vi "DAQ_BlueSteel.vi"() -> ()   [LabVIEW 2016]
uses:
  Control 1.ctl
  <vilib>/DAQmx/write.llb/DAQmx Write (Digital 1D Bool 1Chan 1Samp).vi
  <vilib>/DAQmx/create/channels.llb/DAQmx Create Channel (DO-Digital Output).vi
  <vilib>/DAQmx/miscellaneous.llb/DAQmx Fill In Error Info.vi
  <vilib>/DAQmx/create/channels.llb/DAQmx Create Channel (CO-Pulse Generation-Frequency).vi
  <vilib>/DAQmx/configure/timing.llb/DAQmx Timing (Implicit).vi
  <resource>/objmgr/daqmx.rc
panel:
  out "Ignition":bool
  out "Pump":bool
  out "Record Status":string
  out "TCp-3P Status":bool
  out "TCp-3P":dbl
  out "FM-F Status":bool
  out "FM-F":dbl
  in  "Record":bool
  out "Recording":bool
  out "Solenoid\nStatus":bool[](array[boolean])
  in  "Tab Control":enum32{"Operations", "Testing", "Parameters"}(tab)
  in  "Firing Mode":bool
  in  "Enable Fire Button":bool
  in  "Fuel Arm":bool
  in  "ARM":bool
  in  "ABORT":bool
  out "Arm Indicator":bool
  out "Fuel Arm Indicator 10":bool
  in  "Pressurize":bool
  out "Engine State":string
  out "SAFE":bool
  in  "FIRE":bool
  in  "F Purge":bool
  in  "O Purge":bool
  out "Ox Purged":bool
  out "Fuel Purged":bool
  in  "Depressurize":bool
  out "Fill Volume Bar":dbl(slide) max=258.9 scale=0.0..258.9
  out "Fill Volume (in^3)":dbl
  in  "Manual Fill Reset":bool
  in  "Fuel Prime":bool
  in  "Igniter Prime":bool
  in  "Finish Filling":bool
  in  "Enable Fill Reset":bool
  out "Filled":bool
  in  "Fuel Purge":bool
  in  "Oxygen Purge":bool
  in  "Warning Override":bool
  in  "Spark Safety":bool
  in  "Safety Override":bool[](array[boolean])
  in  "Pump Test":bool
  in  "Spark Test":bool
  in  "NC-P":bool
  in  "NO-P":bool
  in  "NC-F":bool
  in  "NC-O":bool
  in  "NC-IF":bool
  in  "NC-IO":T1
  in  "Parameters":dbl[](array[numeric])
  in  "Max Volume (in^3)":dbl
  in  "Fill Rate (in^3/s)":dbl
  out "PT-TI Status":bool
  out "PT-TI":dbl
  out "PT-IO Status":bool
  out "PT-IO":dbl
  out "FM-O Status":bool
  out "FM-O":dbl
  out "PT-3P Status":bool
  out "PT-3P":dbl
  out "PT-2E Status":bool
  out "PT-2E":dbl
  out "PT-1E Status":bool
  out "PT-1E":dbl
  out "PT-2P Status":bool
  out "PT-2P":dbl
  out "PT-1P Status":bool
  out "PT-1P":dbl
  out "PT-3O Status":bool
  out "PT-3O":dbl
  out "PT-2O Status":bool
  out "PT-2O":dbl
  out "PT-1O Status":bool
  out "PT-1O":dbl
  out "PT-IF Status":bool
  out "PT-IF":dbl
  out "PT-3F Status":bool
  out "PT-3F":dbl
  out "PT-2F Status":bool
  out "PT-2F":dbl
  out "PT-1F Status":bool
  out "PT-1F":dbl
  out "PT-L Status":bool
  out "PT-L":dbl
  out "LC-1E Status":bool
  out "LC-1E":dbl
  out "TCp-2P Status":bool
  out "TCp-2P":dbl
  out "TCp-1P Status":bool
  out "TCp-1P":dbl
  out "TCp-TI Status":bool
  out "TCp-TI":dbl
  out "TCp-2F Status":bool
  out "TCp-2F":dbl
  out "TCp-1F Status":bool
  out "TCp-1F":dbl
  out "TCw-4E Status":bool
  out "TCw-4E":dbl
  out "TCw-3E Status":bool
  out "TCw-3E":dbl
  out "TCw-2E Status":bool
  out "TCw-2E":dbl
  out "TCw-1E Status":bool
  out "TCw-1E":dbl
  out "TCp-3O Status":bool
  out "TCp-3O":dbl
  out "TCp-2O Status":bool
  out "TCp-2O":dbl
  out "TCp-1O Status":bool
  out "TCp-1O":dbl
  # "Red warnings are based on the sensor warning chart in the DAQ project folder on The LPL Drive. A warning will cause an\nautomatic abort on the Operations pane.\n\nThese warnings do not prevent the operation of switches in the Testing pane."
  # "Thermocouples  (F)"
  # "Load Cells (lbf)"
  # "Flow Meters (kg/s)"
  # "Pressure Transducers (psi)"
  # "NC-P"
  # "NO-P"
  # "NC-F"
  # "NC-O"
  # "NC-IF"
  # "NC-IO"
  # "Hot\nFire"
  # "Igniter\nTest"
  # "WARNING: Follow fill procedures to ensure proper\npriming and to avoid fuel waste."
  # "Warning override prevents automatic aborts when\nred flags are active on any sensor readouts."
  # "Safety override is required when PTs on either side of the valve \nread > 100 psid."
  # "Fill Parameters"
  # "Pressurisation P tolerance lower limit (psi)"
  # "Pressurisation P tolerance upper limit (psi)"
  # "Fuel delay (secs)"
  # "Ox delay (secs)"
  # "Spark delay (secs)"
  # "Ignitor pressure threshold (psi)"
  # "Combustion pressure threshold (psi)"
  # "Ignitor run time (secs)"
  # "Engine run time (secs)"
  # "Fuel line pressure threshold (psi)"
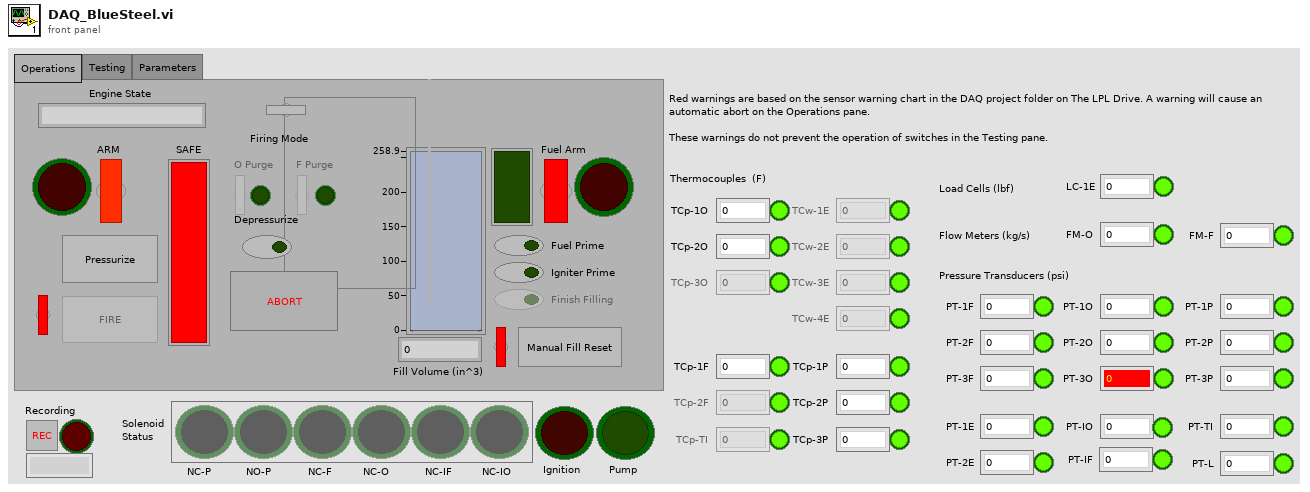
[diagram p1: front panel]
types:
  T1 = typedef "Control 1.ctl" = bool
  T2 = enum8{"Enabled", "Disabled", "Disabled and Grayed Out"}
  T3 = cluster{"[0]":dbl, "[1]":dbl, "[2]":dbl, "[3]":dbl, "[4]":dbl, "[5]":dbl, "[6]":dbl, "[7]":dbl, "[8]":dbl}
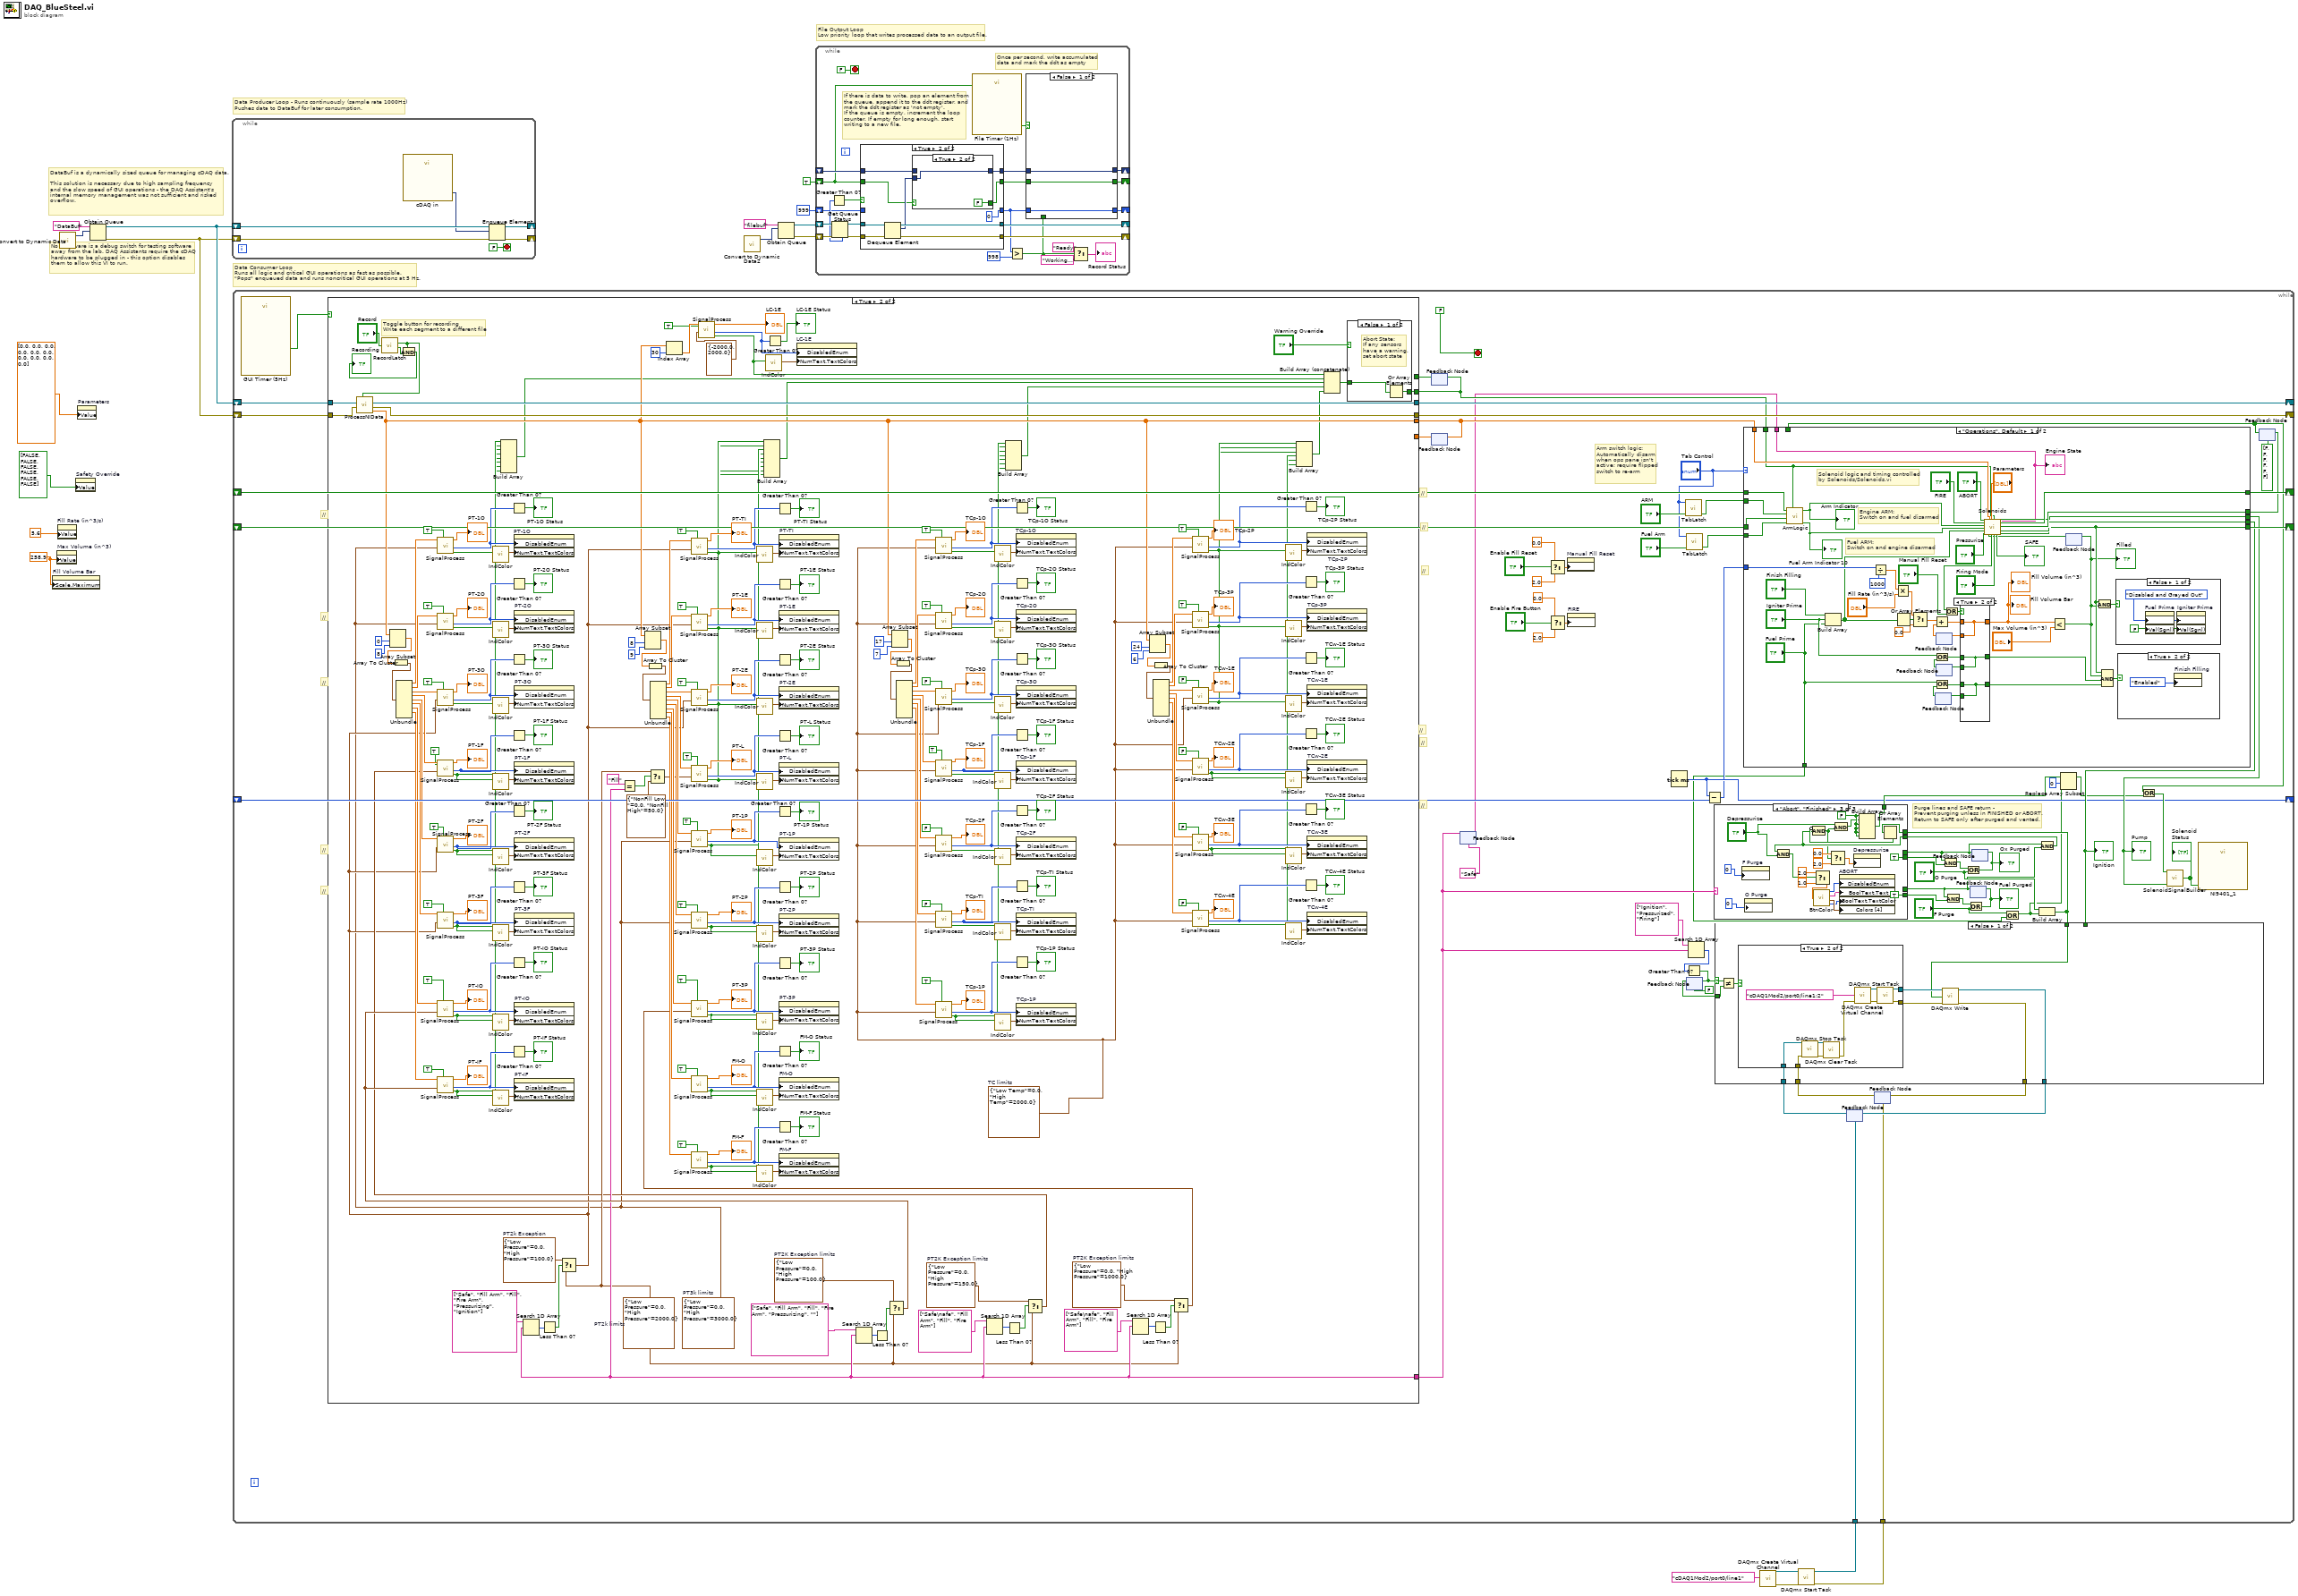
[diagram p0: block diagram]
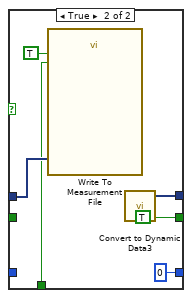
[diagram p2: hidden frame]
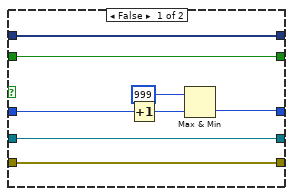
[diagram p3: hidden frame]
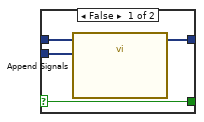
[diagram p4: hidden frame]
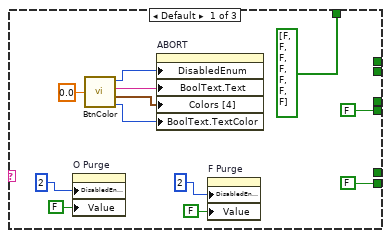
[diagram p5: hidden frame]
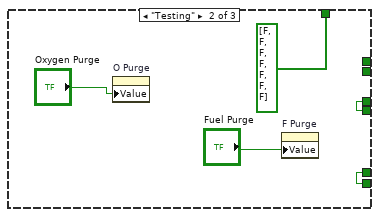
[diagram p6: hidden frame]
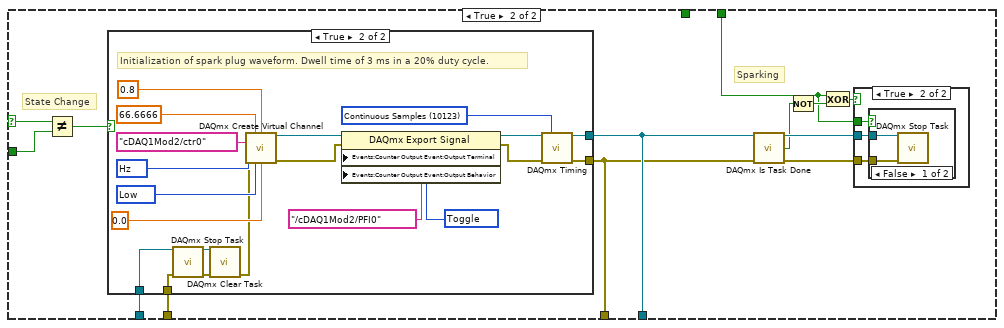
[diagram p8: hidden frame]
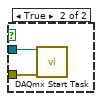
[diagram p10: hidden frame]
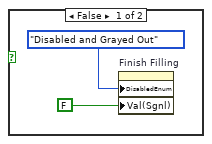
[diagram p12: hidden frame]
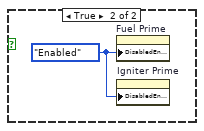
[diagram p13: hidden frame]
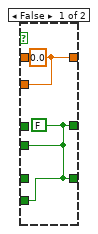
[diagram p14: hidden frame]
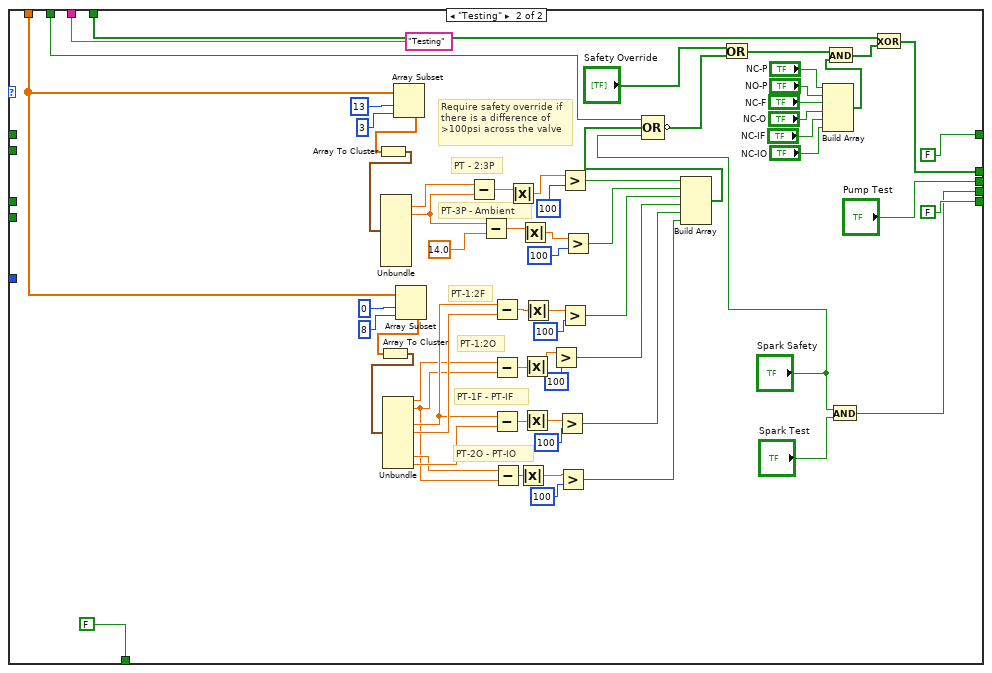
[diagram p15: hidden frame]
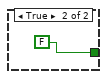
[diagram p17: hidden frame]
diagram:
  w1 = 258.9
  # "File Output Loop\nLow priority loop that writes processed data to an output file."
  # "Data Consumer Loop\nRuns all logic and critical GUI operations as fast as possible.\n\"Pops\" enqueued data and runs noncritical GUI operations at 5 Hz."
  # "No Hardware is a debug switch for testing software\naway from the lab. DAQ Assistants require the cDAQ\nhardware to be plugged in - this option disables \nthem to allow this VI to run."
  # "Data Producer Loop - Runs continuously (sample rate 1000Hz)\nPushes data to DataBuf for later consumption."
  # "DataBuf is a dynamically sized queue for managing cDAQ data.\n\nThis solution is necessary due to high sampling frequency \nand the slow speed of GUI operations - the DAQ Assistant's\ninternal memory management was not sufficient and risked\noverflow."
  n1 = property on="Fill Volume Bar" class="Slide (strict)"("Scale.Maximum"=w1) -> ()  [unwired: 2 in, 2 out]
  n2 = property on="Max Volume (in^3)" class="DigNum (strict)"("Value"=w1) -> ()  [unwired: 2 in, 2 out]
  n3 = property on="Fill Rate (in^3/s)" class="DigNum (strict)"("Value"=5.6) -> ()  [unwired: 2 in, 2 out]
  n4 = call "Convert to Dynamic Data"() -> ("Dynamic Data Type"=w18:dynamicdata)  [unwired: 4 in]
  n5 = property on="Safety Override" class="Arr (strict)"("Value"=bool[] [FALSE, FALSE, FALSE, FALSE, FALSE, FALSE]) -> ()  [unwired: 2 in, 2 out]
  n6 = property on="Parameters" class="Arr (strict)"("Value"=dbl[] [0.0, 0.0, 0.0, 0.0, 0.0, 0.0, 0.0, 0.0, 0.0, 0.0]) -> ()  [unwired: 2 in, 2 out]
  n7 = Obtain Queue(name (unnamed)="DataBuf", element data type=w18) -> (queue out=w17:refnum<queue>, error out=w16:errorcluster)  [unwired: 3 in, 1 out]
  n8 = while {
    shift-right: [w22] -> _
    shift-left: w16 -> [w23]
    shift-right: [w24] -> _
    shift-left: w17 -> [w25]
    stop <- FALSE stop-if-true
    n9 = call "cDAQ in"() -> ("data"=w20:dynamicdata)  [unwired: 16 in, 3 out]
    n10 = Enqueue Element(queue=w25, element=w20, error in (no error)=w23) -> (queue out=w24:refnum<queue>, error out=w22:errorcluster)  [unwired: 1 in, 1 out]
  }
  n11 = call "Convert to Dynamic Data2"() -> ("Dynamic Data Type"=w14:dynamicdata)  [unwired: 4 in]
  n12 = Obtain Queue(name (unnamed)="filebuf", element data type=w14) -> (queue out=w13:refnum<queue>, error out=w12:errorcluster)  [unwired: 3 in, 1 out]
  n13 = while {
    shift-right: [w48] -> _
    shift-left: w12 -> [w40]
    shift-right: [w49] -> _
    shift-left: w13 -> [w41]
    shift-right: [w46] -> _
    shift-left: _ -> [w47]
    shift-right: [w45] -> _
    shift-left: TRUE -> [w34]
    shift-right: [w32] -> _
    shift-left: 999 -> [w33]
    stop <- FALSE stop-if-true
    # "If there is data to write, pop an element from\nthe queue, append it to the ddt register, and\nmark the ddt register as 'not empty'.\nIf the queue is empty, increment the loop\ncounter. If empty for long enough, start\nwriting to a new file."
    # "Once per second, write accumulated\ndata and mark the ddt as empty"
    n14 = Get Queue Status(queue=w41, error in (no error)=w40) -> (queue out=w43:refnum<queue>, error out=w42:errorcluster, # elements in queue=w38:i32)  [unwired: 1 in, 5 out]
    n15 = Greater Than 0?(x=w38) -> (x > 0?=w39:bool)
    n16 = case shown="True" w39 {
      tunnel: w43 -> [w65 w76]
      tunnel: w42 -> [w64 w75]
      tunnel: [w65 w74] -> w49
      tunnel: [w64 w73] -> w48
      tunnel: [w66 w72] -> w37
      tunnel: w47 -> [w66 w70]
      tunnel: w34 -> [w63 w69]
      tunnel: [w63 w68] -> w36
      tunnel: w33 -> [w62 _]
      tunnel: [w59 0] -> w28
      frame False {
        n17 = Increment(x=w62) -> (x+1=w61:i32)
        n18 = Max & Min(x=999, y=w61) -> (min(x,y)=w59:i32)  [unwired: 1 out]
      }
      frame True {
        n19 = Dequeue Element(queue=w76, error in (no error)=w75) -> (queue out=w74:refnum<queue>, element=w71:dynamicdata, error out=w73:errorcluster)  [unwired: 1 in, 1 out]
        n20 = case shown="True" w69 {
          selector: w69 -> [w77 _]
          tunnel: [w80 w82] -> w72
          tunnel: w71 -> [w79 w82]
          tunnel: w70 -> [w78 _]
          tunnel: [w77 FALSE] -> w68
          frame False {
            n21 = call "Append Signals"("Input Signal B"=w79, "Input Signal A"=w78) -> ("Appended Signals"=w80:dynamicdata)  [unwired: 8 in, 1 out]
          }
          frame True {
          }
        }
      }
    }
    n22 = call "File Timer (1Hz)"("Reset"=w34) -> ("Time has Elapsed"=w44:bool)  [unwired: 11 in, 7 out]
    n23 = Greater?(x=w28, y=998) -> (0:w27:bool)
    n24 = case shown="False" w44 {
      tunnel: [w51 w57] -> w46
      tunnel: [w52 TRUE] -> w45
      tunnel: w36 -> [w52 _]
      tunnel: w37 -> [w51 w56]
      tunnel: [w50 0] -> w32
      tunnel: w28 -> [w50 _]
      tunnel: w27 -> [_ w53]
      frame False {
      }
      frame True {
        n25 = call "Write To Measurement File"("Signals"=w56, "Enable"=TRUE, "new_file"=w53) -> ()  [unwired: 14 in, 3 out]
        n26 = call "Convert to Dynamic Data3"() -> ("Dynamic Data Type"=w57:dynamicdata)  [unwired: 4 in]
      }
    }
    n27 = Select(t="Ready", s=w27, f="Working...") -> (s? t:f=→"Record Status":string)
  }
  n28 = call-poly <vilib>:"DAQmx Create Virtual Channel.vi"("lines"=tag "cDAQ1Mod2/port0/line1") -> ("task out"=w8:refnum<k21>, "error out"=w7:errorcluster)  [unwired: 13 in]
  n29 = call <vilib>:"DAQmx Start Task.vi"("task/channels in"=w8, "error in"=w7) -> ("task out"=w6:refnum<k21>, "error out"=w5:errorcluster)  [unwired: 12 in]
  n30 = while {
    shift-right: [w146] -> _
    shift-left: w17 -> [w148]
    shift-right: [w145] -> _
    shift-left: w16 -> [w147]
    shift-right: [w139] -> _
    shift-left: _ -> [w140]
    shift-right: [w137] -> _
    shift-left: _ -> [w138]
    shift-right: [w91] -> _
    shift-left: _ -> [w136]
    tunnel: w6 -> [w114]
    tunnel: w5 -> [w113]
    stop <- FALSE stop-if-true
    # "Purge lines and SAFE return -\nPrevent purging unless in FINISHED or ABORT.\nReturn to SAFE only after purged and vented."
    # "//"
    # "//"
    # "//"
    # "//"
    # "//"
    # "//"
    # "//"
    # "//"
    # "//"
    # "//"
    # "//"
    # "Arm switch logic:\nAutomatically disarm\nwhen ops pane isn't\nactive; require flipped\nswitch to re-arm"
    n31 = call "GUI Timer (5Hz)"() -> ("Time has Elapsed"=w149:bool)  [unwired: 12 in, 7 out]
    n32 = feedback #1() -> (w132:bool)  [unwired: 1 in]
    n33 = feedback #2() -> (w134:dbl[])  [unwired: 1 in]
    n34 = feedback #3("Safe") -> (w108:string)
    n35 = case shown="True" w149 {
      tunnel: w148 -> [w386 w665]
      tunnel: w147 -> [w385 w664]
      tunnel: [w386 w535] -> w146
      tunnel: [w385 w534] -> w145
      tunnel: [w384 w486] -> w131
      tunnel: w134 -> [w384 _]
      tunnel: [w383 w461] -> w133
      tunnel: w132 -> [w383 _]
      tunnel: w108 -> [_ w394]
      frame False {
      }
      frame True {
        w395 = cluster{"Low Pressure":dbl, "High Pressure":dbl} {"Low Pressure"=0.0, "High Pressure"=1000.0}  # PT2K Exception limits
        w399 = cluster{"Low Pressure":dbl, "High Pressure":dbl} {"Low Pressure"=0.0, "High Pressure"=150.0}  # PT2K Exception limits
        w404 = cluster{"Low Pressure":dbl, "High Pressure":dbl} {"Low Pressure"=0.0, "High Pressure"=100.0}  # PT2K Exception limits
        w408 = cluster{"Low Pressure":dbl, "High Pressure":dbl} {"Low Pressure"=0.0, "High Pressure"=100.0}  # PT2k Exception
        w409 = cluster{"Low Temp":dbl, "High Temp":dbl} {"Low Temp"=0.0, "High Temp"=2000.0}  # TC limits
        w388 = cluster{"Low Pressure":dbl, "High Pressure":dbl} {"Low Pressure"=0.0, "High Pressure"=3000.0}  # PT3k limits
        w393 = cluster{"Low Pressure":dbl, "High Pressure":dbl} {"Low Pressure"=0.0, "High Pressure"=2000.0}  # PT2k limits
        # "Toggle button for recording\nWrite each segment to a different file"
        n36 = call "RecordLatch.vi"("Rec Button"="Record") -> ("Indicator"=w532:bool, "Record"=w519:bool)  [unwired: 6 in]
        n37 = call "ProcessNIData.vi"("Record Data"=w519, "Error In"=w664, "Queue In"=w665) -> ("Data Out"=w486:dbl[], "Error Out"=w534:errorcluster, "Queue Out"=w535:refnum<queue>)  [unwired: 6 in]
        n38 = Array Subset(array=w486, index=0, length=8) -> (w611:dbl[])
        n39 = Array To Cluster(array=w611) -> (cluster=w610:T3)
        n40 = Unbundle(w610) -> ("[0]"=w605:dbl, "[1]"=w604:dbl, "[2]"=w603:dbl, "[3]"=w525:dbl, "[4]"=w524:dbl, "[5]"=w523:dbl, "[6]"=w522:dbl, "[7]"=w521:dbl)  [unwired: 1 out]
        n41 = And(x=w519, y=w532) -> (x .and. y?=→"Recording":bool)
        n42 = call "SignalProcess.vi"("Enabled"=TRUE, "Cluster"=w388, "Signal"=w605) -> ("Warning"=w429:bool, "Disable"=w487:i32, "Signal Out"=→"PT-1O":dbl)  [unwired: 6 in]
        n43 = call "SignalProcess.vi"("Enabled"=TRUE, "Cluster"=w388, "Signal"=w604) -> ("Warning"=w428:bool, "Disable"=w656:i32, "Signal Out"=→"PT-2O":dbl)  [unwired: 6 in]
        n44 = call "IndColor.vi"("Warning"=w429) -> ("IndColor"=w430:cluster{"BGColor":dbl, "TextColor":dbl})  [unwired: 10 in]
        n45 = call "IndColor.vi"("Warning"=w428) -> ("IndColor"=w431:cluster{"BGColor":dbl, "TextColor":dbl})  [unwired: 10 in]
        n46 = Greater Than 0?(x=w487) -> (x > 0?=→"PT-1O Status":bool)
        n47 = Greater Than 0?(x=w656) -> (x > 0?=→"PT-2O Status":bool)
        n48 = property on="PT-1O" class="DigNum (strict)"("DisabledEnum"=w487, "NumText.TextColors"=w430) -> ()  [unwired: 2 in, 2 out]
        n49 = property on="PT-2O" class="DigNum (strict)"("DisabledEnum"=w656, "NumText.TextColors"=w431) -> ()  [unwired: 2 in, 2 out]
        n50 = Search 1D Array(1D array=string[] ["Safe", "Fill Arm", "Fill", "Fire Arm", "Pressurizing", "Ignition"], element=w394) -> (index of element=w411:i32)  [unwired: 1 in]
        n51 = Less Than 0?(x=w411) -> (x < 0?=w410:bool)
        n52 = Select(t=w408, s=w410, f=w393) -> (s? t:f=w389:cluster{"Low Pressure":dbl, "High Pressure":dbl})
        n53 = call "SignalProcess.vi"("Enabled"=TRUE, "Cluster"=w389, "Signal"=w603) -> ("Warning"=w427:bool, "Disable"=w654:i32, "Signal Out"=→"PT-3O":dbl)  [unwired: 6 in]
        n54 = call "SignalProcess.vi"("Enabled"=TRUE, "Cluster"=w389, "Signal"=w524) -> ("Warning"=w425:bool, "Disable"=w647:i32, "Signal Out"=→"PT-2F":dbl)  [unwired: 6 in]
        n55 = call "SignalProcess.vi"("Enabled"=TRUE, "Cluster"=w389, "Signal"=w523) -> ("Warning"=w424:bool, "Disable"=w645:i32, "Signal Out"=→"PT-3F":dbl)  [unwired: 6 in]
        n56 = call "IndColor.vi"("Warning"=w427) -> ("IndColor"=w432:cluster{"BGColor":dbl, "TextColor":dbl})  [unwired: 10 in]
        n57 = call "IndColor.vi"("Warning"=w425) -> ("IndColor"=w434:cluster{"BGColor":dbl, "TextColor":dbl})  [unwired: 10 in]
        n58 = call "IndColor.vi"("Warning"=w424) -> ("IndColor"=w435:cluster{"BGColor":dbl, "TextColor":dbl})  [unwired: 10 in]
        n59 = Greater Than 0?(x=w654) -> (x > 0?=→"PT-3O Status":bool)
        n60 = Greater Than 0?(x=w647) -> (x > 0?=→"PT-2F Status":bool)
        n61 = Greater Than 0?(x=w645) -> (x > 0?=→"PT-3F Status":bool)
        n62 = property on="PT-3O" class="DigNum (strict)"("DisabledEnum"=w654, "NumText.TextColors"=w432) -> ()  [unwired: 2 in, 2 out]
        n63 = property on="PT-2F" class="DigNum (strict)"("DisabledEnum"=w647, "NumText.TextColors"=w434) -> ()  [unwired: 2 in, 2 out]
        n64 = property on="PT-3F" class="DigNum (strict)"("DisabledEnum"=w645, "NumText.TextColors"=w435) -> ()  [unwired: 2 in, 2 out]
        n65 = Equal?(x="Fill", y=w394) -> (x = y?=w415:bool)
        n66 = Array Subset(array=w486, index=8, length=9) -> (w607:dbl[])
        n67 = Array To Cluster(array=w607) -> (cluster=w606:T3)
        n68 = Select(t=w393, s=w415, f=cluster{"NonFill Low ":dbl, "NonFill High":dbl} {"NonFill Low "=0.0, "NonFill High"=50.0}) -> (s? t:f=w416:cluster{"NonFill Low ":dbl, "NonFill High":dbl})
        n69 = Unbundle(w606) -> ("[0]"=w526:dbl, "[1]"=w602:dbl, "[2]"=w601:dbl, "[3]"=w600:dbl, "[4]"=w599:dbl, "[5]"=w598:dbl, "[6]"=w597:dbl, "[7]"=w530:dbl, "[8]"=w520:dbl)
        n70 = Index Array(array=w486, index=30) -> (element=w592:dbl)
        n71 = call "SignalProcess.vi"("Enabled"=TRUE, "Cluster"=w389, "Signal"=w526) -> ("Warning"=w445:bool, "Disable"=w636:i32, "Signal Out"=→"PT-TI":dbl)  [unwired: 6 in]
        n72 = call "SignalProcess.vi"("Enabled"=TRUE, "Cluster"=w389, "Signal"=w602) -> ("Warning"=w446:bool, "Disable"=w633:i32, "Signal Out"=→"PT-1E":dbl)  [unwired: 6 in]
        n73 = call "SignalProcess.vi"("Enabled"=TRUE, "Cluster"=w389, "Signal"=w601) -> ("Warning"=w438:bool, "Disable"=w630:i32, "Signal Out"=→"PT-2E":dbl)  [unwired: 6 in]
        n74 = call "SignalProcess.vi"("Enabled"=TRUE, "Cluster"=w416, "Signal"=w600) -> ("Warning"=w439:bool, "Disable"=w627:i32, "Signal Out"=→"PT-L":dbl)  [unwired: 6 in]
        n75 = call "SignalProcess.vi"("Enabled"=TRUE, "Cluster"=w388, "Signal"=w599) -> ("Warning"=w440:bool, "Disable"=w624:i32, "Signal Out"=→"PT-1P":dbl)  [unwired: 6 in]
        n76 = call "SignalProcess.vi"("Enabled"=TRUE, "Cluster"=w388, "Signal"=w598) -> ("Warning"=w441:bool, "Disable"=w621:i32, "Signal Out"=→"PT-2P":dbl)  [unwired: 6 in]
        n77 = call "SignalProcess.vi"("Enabled"=TRUE, "Signal"=w530) -> ("Warning"=w443:bool, "Disable"=w614:i32, "Signal Out"=→"FM-O":dbl)  [unwired: 7 in]
        n78 = call "SignalProcess.vi"("Enabled"=TRUE, "Signal"=w520) -> ("Warning"=w444:bool, "Disable"=w594:i32, "Signal Out"=→"FM-F":dbl)  [unwired: 7 in]
        n79 = call "SignalProcess.vi"("Enabled"=TRUE, "Cluster"=cluster{dbl, dbl} {-2000.0, 2000.0}, "Signal"=w592) -> ("Warning"=w417:bool, "Disable"=w662:i32, "Signal Out"=→"LC-1E":dbl)  [unwired: 6 in]
        n80 = call "IndColor.vi"("Warning"=w445) -> ("IndColor"=w462:cluster{"BGColor":dbl, "TextColor":dbl})  [unwired: 10 in]
        n81 = call "IndColor.vi"("Warning"=w446) -> ("IndColor"=w463:cluster{"BGColor":dbl, "TextColor":dbl})  [unwired: 10 in]
        n82 = call "IndColor.vi"("Warning"=w438) -> ("IndColor"=w464:cluster{"BGColor":dbl, "TextColor":dbl})  [unwired: 10 in]
        n83 = call "IndColor.vi"("Warning"=w439) -> ("IndColor"=w465:cluster{"BGColor":dbl, "TextColor":dbl})  [unwired: 10 in]
        n84 = call "IndColor.vi"("Warning"=w440) -> ("IndColor"=w466:cluster{"BGColor":dbl, "TextColor":dbl})  [unwired: 10 in]
        n85 = call "IndColor.vi"("Warning"=w441) -> ("IndColor"=w467:cluster{"BGColor":dbl, "TextColor":dbl})  [unwired: 10 in]
        n86 = call "IndColor.vi"("Warning"=w443) -> ("IndColor"=w469:cluster{"BGColor":dbl, "TextColor":dbl})  [unwired: 10 in]
        n87 = call "IndColor.vi"("Warning"=w444) -> ("IndColor"=w470:cluster{"BGColor":dbl, "TextColor":dbl})  [unwired: 10 in]
        n88 = call "IndColor.vi"("Warning"=w417) -> ("IndColor"=w471:cluster{"BGColor":dbl, "TextColor":dbl})  [unwired: 10 in]
        n89 = Greater Than 0?(x=w662) -> (x > 0?=→"LC-1E Status":bool)
        n90 = Greater Than 0?(x=w636) -> (x > 0?=→"PT-TI Status":bool)
        n91 = Greater Than 0?(x=w633) -> (x > 0?=→"PT-1E Status":bool)
        n92 = Greater Than 0?(x=w630) -> (x > 0?=→"PT-2E Status":bool)
        n93 = Greater Than 0?(x=w627) -> (x > 0?=→"PT-L Status":bool)
        n94 = Greater Than 0?(x=w624) -> (x > 0?=→"PT-1P Status":bool)
        n95 = Greater Than 0?(x=w621) -> (x > 0?=→"PT-2P Status":bool)
        n96 = Greater Than 0?(x=w614) -> (x > 0?=→"FM-O Status":bool)
        n97 = Greater Than 0?(x=w594) -> (x > 0?=→"FM-F Status":bool)
        n98 = property on="PT-TI" class="DigNum (strict)"("DisabledEnum"=w636, "NumText.TextColors"=w462) -> ()  [unwired: 2 in, 2 out]
        n99 = property on="PT-1E" class="DigNum (strict)"("DisabledEnum"=w633, "NumText.TextColors"=w463) -> ()  [unwired: 2 in, 2 out]
        n100 = property on="PT-2E" class="DigNum (strict)"("DisabledEnum"=w630, "NumText.TextColors"=w464) -> ()  [unwired: 2 in, 2 out]
        n101 = property on="PT-L" class="DigNum (strict)"("DisabledEnum"=w627, "NumText.TextColors"=w465) -> ()  [unwired: 2 in, 2 out]
        n102 = property on="PT-1P" class="DigNum (strict)"("DisabledEnum"=w624, "NumText.TextColors"=w466) -> ()  [unwired: 2 in, 2 out]
        n103 = property on="PT-2P" class="DigNum (strict)"("DisabledEnum"=w621, "NumText.TextColors"=w467) -> ()  [unwired: 2 in, 2 out]
        n104 = property on="FM-O" class="DigNum (strict)"("DisabledEnum"=w614, "NumText.TextColors"=w469) -> ()  [unwired: 2 in, 2 out]
        n105 = property on="FM-F" class="DigNum (strict)"("DisabledEnum"=w594, "NumText.TextColors"=w470) -> ()  [unwired: 2 in, 2 out]
        n106 = property on="LC-1E" class="DigNum (strict)"("DisabledEnum"=w662, "NumText.TextColors"=w471) -> ()  [unwired: 2 in, 2 out]
        n107 = Search 1D Array(1D array=string[] ["Safe", "Fill Arm", "Fill", "Fire Arm", "Pressurizing", ""], element=w394) -> (index of element=w406:i32)  [unwired: 1 in]
        n108 = Less Than 0?(x=w406) -> (x < 0?=w405:bool)
        n109 = Select(t=w404, s=w405, f=w393) -> (s? t:f=w403:cluster{"Low Pressure":dbl, "High Pressure":dbl})
        n110 = call "SignalProcess.vi"("Enabled"=TRUE, "Cluster"=w403, "Signal"=w522) -> ("Warning"=w423:bool, "Disable"=w641:i32, "Signal Out"=→"PT-IO":dbl)  [unwired: 6 in]
        n111 = call "SignalProcess.vi"("Enabled"=TRUE, "Cluster"=w403, "Signal"=w521) -> ("Warning"=w422:bool, "Disable"=w639:i32, "Signal Out"=→"PT-IF":dbl)  [unwired: 6 in]
        n112 = call "IndColor.vi"("Warning"=w423) -> ("IndColor"=w436:cluster{"BGColor":dbl, "TextColor":dbl})  [unwired: 10 in]
        n113 = call "IndColor.vi"("Warning"=w422) -> ("IndColor"=w437:cluster{"BGColor":dbl, "TextColor":dbl})  [unwired: 10 in]
        n114 = Greater Than 0?(x=w641) -> (x > 0?=→"PT-IO Status":bool)
        n115 = Greater Than 0?(x=w639) -> (x > 0?=→"PT-IF Status":bool)
        n116 = property on="PT-IO" class="DigNum (strict)"("DisabledEnum"=w641, "NumText.TextColors"=w436) -> ()  [unwired: 2 in, 2 out]
        n117 = property on="PT-IF" class="DigNum (strict)"("DisabledEnum"=w639, "NumText.TextColors"=w437) -> ()  [unwired: 2 in, 2 out]
        n118 = Array Subset(array=w486, index=17, length=7) -> (w589:dbl[])
        n119 = Array To Cluster(array=w589) -> (cluster=w588:T3)
        n120 = Unbundle(w588) -> ("[0]"=w566:dbl, "[1]"=w565:dbl, "[2]"=w564:dbl, "[3]"=w485:dbl, "[4]"=w529:dbl, "[5]"=w528:dbl, "[6]"=w527:dbl)  [unwired: 2 out]
        n121 = call "SignalProcess.vi"("Enabled"=TRUE, "Cluster"=w409, "Signal"=w566) -> ("Warning"=w453:bool, "Disable"=w586:i32, "Signal Out"=→"TCp-1O":dbl)  [unwired: 6 in]
        n122 = call "SignalProcess.vi"("Enabled"=TRUE, "Cluster"=w409, "Signal"=w565) -> ("Warning"=w452:bool, "Disable"=w583:i32, "Signal Out"=→"TCp-2O":dbl)  [unwired: 6 in]
        n123 = call "SignalProcess.vi"("Enabled"=FALSE, "Cluster"=w409, "Signal"=w564) -> ("Warning"=w451:bool, "Disable"=w580:i32, "Signal Out"=→"TCp-3O":dbl)  [unwired: 6 in]
        n124 = call "SignalProcess.vi"("Enabled"=TRUE, "Cluster"=w409, "Signal"=w485) -> ("Warning"=w450:bool, "Disable"=w577:i32, "Signal Out"=→"TCp-1F":dbl)  [unwired: 6 in]
        n125 = call "SignalProcess.vi"("Enabled"=FALSE, "Cluster"=w409, "Signal"=w529) -> ("Warning"=w449:bool, "Disable"=w574:i32, "Signal Out"=→"TCp-2F":dbl)  [unwired: 6 in]
        n126 = call "SignalProcess.vi"("Enabled"=FALSE, "Cluster"=w409, "Signal"=w528) -> ("Warning"=w448:bool, "Disable"=w571:i32, "Signal Out"=→"TCp-TI":dbl)  [unwired: 6 in]
        n127 = call "SignalProcess.vi"("Enabled"=TRUE, "Cluster"=w409, "Signal"=w527) -> ("Warning"=w447:bool, "Disable"=w568:i32, "Signal Out"=→"TCp-1P":dbl)  [unwired: 6 in]
        n128 = Search 1D Array(1D array=string[] ["Safe\nafe", "Fill Arm", "Fill", "Fire Arm"] ("String"), element=w394) -> (index of element=w401:i32)  [unwired: 1 in]
        n129 = call "IndColor.vi"("Warning"=w453) -> ("IndColor"=w472:cluster{"BGColor":dbl, "TextColor":dbl})  [unwired: 10 in]
        n130 = call "IndColor.vi"("Warning"=w452) -> ("IndColor"=w473:cluster{"BGColor":dbl, "TextColor":dbl})  [unwired: 10 in]
        n131 = call "IndColor.vi"("Warning"=w451) -> ("IndColor"=w474:cluster{"BGColor":dbl, "TextColor":dbl})  [unwired: 10 in]
        n132 = call "IndColor.vi"("Warning"=w450) -> ("IndColor"=w475:cluster{"BGColor":dbl, "TextColor":dbl})  [unwired: 10 in]
        n133 = call "IndColor.vi"("Warning"=w449) -> ("IndColor"=w476:cluster{"BGColor":dbl, "TextColor":dbl})  [unwired: 10 in]
        n134 = call "IndColor.vi"("Warning"=w448) -> ("IndColor"=w477:cluster{"BGColor":dbl, "TextColor":dbl})  [unwired: 10 in]
        n135 = call "IndColor.vi"("Warning"=w447) -> ("IndColor"=w478:cluster{"BGColor":dbl, "TextColor":dbl})  [unwired: 10 in]
        n136 = Build Array(w453, w452, w451, w450, w449, w448, w447) -> (w420:bool[])
        n137 = Less Than 0?(x=w401) -> (x < 0?=w400:bool)
        n138 = Greater Than 0?(x=w586) -> (x > 0?=→"TCp-1O Status":bool)
        n139 = Greater Than 0?(x=w583) -> (x > 0?=→"TCp-2O Status":bool)
        n140 = Greater Than 0?(x=w580) -> (x > 0?=→"TCp-3O Status":bool)
        n141 = Greater Than 0?(x=w577) -> (x > 0?=→"TCp-1F Status":bool)
        n142 = Greater Than 0?(x=w574) -> (x > 0?=→"TCp-2F Status":bool)
        n143 = Greater Than 0?(x=w571) -> (x > 0?=→"TCp-TI Status":bool)
        n144 = Greater Than 0?(x=w568) -> (x > 0?=→"TCp-1P Status":bool)
        n145 = property on="TCp-1O" class="DigNum (strict)"("DisabledEnum"=w586, "NumText.TextColors"=w472) -> ()  [unwired: 2 in, 2 out]
        n146 = property on="TCp-2O" class="DigNum (strict)"("DisabledEnum"=w583, "NumText.TextColors"=w473) -> ()  [unwired: 2 in, 2 out]
        n147 = property on="TCp-3O" class="DigNum (strict)"("DisabledEnum"=w580, "NumText.TextColors"=w474) -> ()  [unwired: 2 in, 2 out]
        n148 = property on="TCp-1F" class="DigNum (strict)"("DisabledEnum"=w577, "NumText.TextColors"=w475) -> ()  [unwired: 2 in, 2 out]
        n149 = property on="TCp-2F" class="DigNum (strict)"("DisabledEnum"=w574, "NumText.TextColors"=w476) -> ()  [unwired: 2 in, 2 out]
        n150 = property on="TCp-TI" class="DigNum (strict)"("DisabledEnum"=w571, "NumText.TextColors"=w477) -> ()  [unwired: 2 in, 2 out]
        n151 = property on="TCp-1P" class="DigNum (strict)"("DisabledEnum"=w568, "NumText.TextColors"=w478) -> ()  [unwired: 2 in, 2 out]
        n152 = Select(t=w399, s=w400, f=w393) -> (s? t:f=w392:cluster{"Low Pressure":dbl, "High Pressure":dbl})
        n153 = call "SignalProcess.vi"("Enabled"=TRUE, "Cluster"=w392, "Signal"=w525) -> ("Warning"=w426:bool, "Disable"=w650:i32, "Signal Out"=→"PT-1F":dbl)  [unwired: 6 in]
        n154 = call "IndColor.vi"("Warning"=w426) -> ("IndColor"=w433:cluster{"BGColor":dbl, "TextColor":dbl})  [unwired: 10 in]
        n155 = Build Array(w429, w428, w427, w426, w425, w424, w423, w422) -> (w418:bool[])
        n156 = Greater Than 0?(x=w650) -> (x > 0?=→"PT-1F Status":bool)
        n157 = property on="PT-1F" class="DigNum (strict)"("DisabledEnum"=w650, "NumText.TextColors"=w433) -> ()  [unwired: 2 in, 2 out]
        n158 = Search 1D Array(1D array=string[] ["Safe\nafe", "Fill Arm", "Fill", "Fire Arm"] ("String"), element=w394) -> (index of element=w397:i32)  [unwired: 1 in]
        n159 = Array Subset(array=w486, index=24, length=6) -> (w543:dbl[])
        n160 = Less Than 0?(x=w397) -> (x < 0?=w396:bool)
        n161 = Array To Cluster(array=w543) -> (cluster=w542:T3)
        n162 = Unbundle(w542) -> ("[0]"=w541:dbl, "[1]"=w540:dbl, "[2]"=w539:dbl, "[3]"=w538:dbl, "[4]"=w537:dbl, "[5]"=w536:dbl)  [unwired: 3 out]
        n163 = Select(t=w395, s=w396, f=w393) -> (s? t:f=w391:cluster{"Low Pressure":dbl, "High Pressure":dbl})
        n164 = call "SignalProcess.vi"("Enabled"=TRUE, "Cluster"=w391, "Signal"=w597) -> ("Warning"=w442:bool, "Disable"=w618:i32, "Signal Out"=→"PT-3P":dbl)  [unwired: 6 in]
        n165 = call "IndColor.vi"("Warning"=w442) -> ("IndColor"=w468:cluster{"BGColor":dbl, "TextColor":dbl})  [unwired: 10 in]
        n166 = Build Array(w446, w445, w444, w443, w442, w441, w440, w439, w438) -> (w419:bool[])
        n167 = Greater Than 0?(x=w618) -> (x > 0?=→"PT-3P Status":bool)
        n168 = property on="PT-3P" class="DigNum (strict)"("DisabledEnum"=w618, "NumText.TextColors"=w468) -> ()  [unwired: 2 in, 2 out]
        n169 = call "SignalProcess.vi"("Enabled"=TRUE, "Cluster"=w409, "Signal"=w541) -> ("Warning"=w459:bool, "Disable"=w562:i32, "Signal Out"=→"TCp-2P":dbl)  [unwired: 6 in]
        n170 = call "SignalProcess.vi"("Enabled"=TRUE, "Cluster"=w409, "Signal"=w540) -> ("Warning"=w458:bool, "Disable"=w547:i32, "Signal Out"=→"TCp-3P":dbl)  [unwired: 6 in]
        n171 = call "SignalProcess.vi"("Enabled"=FALSE, "Cluster"=w409, "Signal"=w539) -> ("Warning"=w457:bool, "Disable"=w559:i32, "Signal Out"=→"TCw-1E":dbl)  [unwired: 6 in]
        n172 = call "SignalProcess.vi"("Enabled"=FALSE, "Cluster"=w409, "Signal"=w538) -> ("Warning"=w456:bool, "Disable"=w556:i32, "Signal Out"=→"TCw-2E":dbl)  [unwired: 6 in]
        n173 = call "SignalProcess.vi"("Enabled"=FALSE, "Cluster"=w409, "Signal"=w537) -> ("Warning"=w455:bool, "Disable"=w553:i32, "Signal Out"=→"TCw-3E":dbl)  [unwired: 6 in]
        n174 = call "SignalProcess.vi"("Enabled"=FALSE, "Cluster"=w409, "Signal"=w536) -> ("Warning"=w454:bool, "Disable"=w550:i32, "Signal Out"=→"TCw-4E":dbl)  [unwired: 6 in]
        n175 = call "IndColor.vi"("Warning"=w459) -> ("IndColor"=w479:cluster{"BGColor":dbl, "TextColor":dbl})  [unwired: 10 in]
        n176 = call "IndColor.vi"("Warning"=w458) -> ("IndColor"=w480:cluster{"BGColor":dbl, "TextColor":dbl})  [unwired: 10 in]
        n177 = call "IndColor.vi"("Warning"=w457) -> ("IndColor"=w481:cluster{"BGColor":dbl, "TextColor":dbl})  [unwired: 10 in]
        n178 = call "IndColor.vi"("Warning"=w456) -> ("IndColor"=w482:cluster{"BGColor":dbl, "TextColor":dbl})  [unwired: 10 in]
        n179 = call "IndColor.vi"("Warning"=w455) -> ("IndColor"=w483:cluster{"BGColor":dbl, "TextColor":dbl})  [unwired: 10 in]
        n180 = call "IndColor.vi"("Warning"=w454) -> ("IndColor"=w484:cluster{"BGColor":dbl, "TextColor":dbl})  [unwired: 10 in]
        n181 = Build Array(w459, w458, w457, w456, w455, w454) -> (w421:bool[])
        n182 = Greater Than 0?(x=w562) -> (x > 0?=→"TCp-2P Status":bool)
        n183 = Greater Than 0?(x=w547) -> (x > 0?=→"TCp-3P Status":bool)
        n184 = Greater Than 0?(x=w559) -> (x > 0?=→"TCw-1E Status":bool)
        n185 = Greater Than 0?(x=w556) -> (x > 0?=→"TCw-2E Status":bool)
        n186 = Greater Than 0?(x=w553) -> (x > 0?=→"TCw-3E Status":bool)
        n187 = Greater Than 0?(x=w550) -> (x > 0?=→"TCw-4E Status":bool)
        n188 = property on="TCp-2P" class="DigNum (strict)"("DisabledEnum"=w562, "NumText.TextColors"=w479) -> ()  [unwired: 2 in, 2 out]
        n189 = property on="TCp-3P" class="DigNum (strict)"("DisabledEnum"=w547, "NumText.TextColors"=w480) -> ()  [unwired: 2 in, 2 out]
        n190 = property on="TCw-1E" class="DigNum (strict)"("DisabledEnum"=w559, "NumText.TextColors"=w481) -> ()  [unwired: 2 in, 2 out]
        n191 = property on="TCw-2E" class="DigNum (strict)"("DisabledEnum"=w556, "NumText.TextColors"=w482) -> ()  [unwired: 2 in, 2 out]
        n192 = property on="TCw-3E" class="DigNum (strict)"("DisabledEnum"=w553, "NumText.TextColors"=w483) -> ()  [unwired: 2 in, 2 out]
        n193 = property on="TCw-4E" class="DigNum (strict)"("DisabledEnum"=w550, "NumText.TextColors"=w484) -> ()  [unwired: 2 in, 2 out]
        n194 = Build Array (concatenate)(w417, w418, w419, w420, w421) -> (w460:bool[])
        n195 = case shown="False" "Warning Override" {
          tunnel: [w667 FALSE] -> w461
          tunnel: w460 -> [w666 _]
          frame False {
            # "Abort State:\nIf any sensors\nhave a warning,\nset abort state"
            n196 = Or Array Elements(Boolean array=w666) -> (logical OR=w667:bool)
          }
          frame True {
          }
        }
      }
    }
    n197 = feedback-in #1(w133) -> ()
    n198 = feedback-in #2(w131) -> ()
    n199 = Select(t=0.0, s="Enable Fill Reset", f=2.0) -> (s? t:f=w87:dbl)
    n200 = Select(t=0.0, s="Enable Fire Button", f=2.0) -> (s? t:f=w125:dbl)
    n201 = property on="Manual Fill Reset" class="Bool (strict)"("DisabledEnum"=w87) -> ()  [unwired: 2 in, 2 out]
    n202 = property on="FIRE" class="Bool"("DisabledEnum"=w125) -> ()  [unwired: 2 in, 2 out]
    n203 = Tick Count (ms)() -> (millisecond timer value=w91:u32)
    n204 = call "TabLatch.vi"("Switch State"="ARM", "Controls Tab"="Tab Control") -> ("Switch State"=w143:bool)  [unwired: 9 in]
    n205 = feedback #4(FALSE) -> (w111:bool)
    n206 = call "TabLatch.vi"("Switch State"="Fuel Arm", "Controls Tab"="Tab Control") -> ("Switch State"=w144:bool)  [unwired: 9 in]
    n207 = Search 1D Array(1D array=string[] ["Ignition", "Pressurized", "Firing"], element=w108) -> (index of element=w120:i32)  [unwired: 1 in]
    n208 = Greater Than 0?(x=w120) -> (x > 0?=w109:bool)
    n209 = feedback-in #4(w109) -> ()
    n210 = Subtract(x=w91, y=w136) -> (x-y=w90:u32)
    n211 = feedback #5(w114) -> (w115:refnum<k21>)
    n212 = feedback #6(w113) -> (w117:errorcluster)
    n213 = feedback #7() -> (w92:bool)  [unwired: 1 in]
    n214 = feedback #8() -> (w93:bool)  [unwired: 1 in]
    n215 = And(x=w93, y=w92) -> (x .and. y?=w100:bool)
    n216 = feedback #9(bool[] [FALSE, FALSE, FALSE, FALSE, FALSE, FALSE]) -> (w98:T1[])
    n217 = case shown="\"Operations\", Default" "Tab Control" {
      tunnel: [w296 FALSE] -> w137
      tunnel: [w262 FALSE] -> w139
      tunnel: w143 -> [w305 _]
      tunnel: w144 -> [w304 _]
      tunnel: w138 -> [w306 _]
      tunnel: w140 -> [w303 _]
      tunnel: [w294 "Pump Test"] -> w122
      tunnel: [w295 w348] -> w135
      tunnel: [w292 w321] -> w112
      tunnel: w131 -> [w297 w357]
      tunnel: w98 -> [_ w349]
      tunnel: w133 -> [w267 w333]
      tunnel: [w290 "Testing"] -> w129
      tunnel: w90 -> [w281 _]
      tunnel: ["Fuel Prime" FALSE] -> w83
      frame "Operations", Default {
        # "Solenoid logic and timing controlled\nby Solenoids/Solenoids.vi"
        # "Fuel ARM:\nSwitch on and engine disarmed"
        # "Engine ARM:\nSwitch on and fuel disarmed"
        n218 = call "ArmLogic.vi"("SensorError"=w267, "FuelArmSwitch"=w304, "PreviousFuelArm"=w303, "ArmSwitch"=w305, "PreviousArm"=w306) -> ("FuelArm"=w293:bool, "Arm"=w300:bool)  [unwired: 5 in]
        "Fuel Arm Indicator 10" <- w293
        "Arm Indicator" <- w300
        n219 = Build Array("Finish Filling", "Igniter Prime", "Fuel Prime") -> (w259:bool[])
        n220 = Divide(x=w281, y=1000) -> (x/y=w283:dbl)
        n221 = Multiply(x=w283, y="Fill Rate (in^3/s)") -> (x*y=w285:dbl)
        n222 = Or Array Elements(Boolean array=w259) -> (logical OR=w287:bool)
        n223 = Select(t=w285, s=w287, f=0.0) -> (s? t:f=w280:dbl)
        n224 = feedback #10() -> (w277:bool)  [unwired: 1 in]
        n225 = Or(x="Fuel Prime", y=w277) -> (x .or. y?=w271:bool)
        n226 = feedback #11() -> (w278:bool)  [unwired: 1 in]
        n227 = Or(x="Igniter Prime", y=w278) -> (x .or. y?=w273:bool)
        n228 = feedback #12() -> (w279:dbl)  [unwired: 1 in]
        n229 = Add(x=w280, y=w279) -> (x+y=w275:dbl)
        n230 = feedback #13() -> (w257:bool)  [unwired: 1 in]
        n231 = call "Solenoids.vi"("Abort Command"="ABORT", "Fire Command"="FIRE", "Fire Arm"=w300, "Fill Arm"=w293, "Fill commands"=w259, "Pressurize command"="Pressurize", "Sensor Data"=w297, "Filled In"=w257, "Parameters"="Parameters", "Sensor Warning"=w267, "Ignition test"="Firing Mode") -> ("Reset Fill Amt"=w258:bool, "Safe"=→"SAFE":bool, "Current State"=w290:string, "Fire Arm Out"=w296:bool, "Valves"=w295:bool[], "Fuel Pump"=w294:bool, "Spark Plug"=w292:bool, "Fill Arm Out"=w262:bool)  [unwired: 1 out]
        "Engine State" <- w290
        n232 = Or(x=w258, y="Manual Fill Reset") -> (x .or. y?=w261:bool)
        n233 = case shown="True" w261 {
          tunnel: [w314 w317] -> w269
          tunnel: w275 -> [_ w317]
          tunnel: [w314 w317] -> w274
          tunnel: [w313 w316] -> w264
          tunnel: w273 -> [_ w316]
          tunnel: [w313 w316] -> w272
          tunnel: [w313 w315] -> w265
          tunnel: w271 -> [_ w315]
          tunnel: [w313 w315] -> w270
          frame False {
            w313 = FALSE
            w314 = 0.0
          }
          frame True {
          }
        }
        "Fill Volume (in^3)" <- w269
        "Fill Volume Bar" <- w269
        n234 = feedback-in #10(w270) -> ()
        n235 = feedback-in #11(w272) -> ()
        n236 = feedback-in #12(w274) -> ()
        n237 = Less?(x=w269, y="Max Volume (in^3)") -> (x < y?=w255:bool)
        "Filled" <- w255
        n238 = feedback-in #13(w255) -> ()
        n239 = Compound Arithmetic op=AND(w262, w255) -> (w266:bool)
        n240 = Compound Arithmetic op=AND(w262, w255, w264, w265) -> (w263:bool)
        n241 = case shown="False" w266 {
          frame False {
            w311 = T2."Disabled and Grayed Out" ("Disabled")
            w310 = FALSE ("Value (Signaling)")
            n242 = property on="Fuel Prime" class="Bool (strict)"("DisabledEnum"=w311, "Val(Sgnl)"=w310) -> ()  [unwired: 2 in, 2 out]
            n243 = property on="Igniter Prime" class="Bool (strict)"("DisabledEnum"=w311, "Val(Sgnl)"=w310) -> ()  [unwired: 2 in, 2 out]
          }
          frame True {
            w312 = T2."Enabled" ("Disabled")
            n244 = property on="Fuel Prime" class="Bool (strict)"("DisabledEnum"=w312) -> ()  [unwired: 2 in, 2 out]
            n245 = property on="Igniter Prime" class="Bool (strict)"("DisabledEnum"=w312) -> ()  [unwired: 2 in, 2 out]
          }
        }
        n246 = case shown="True" w263 {
          frame False {
            n247 = property on="Finish Filling" class="Bool (strict)"("DisabledEnum"=T2."Disabled and Grayed Out" ("Disabled"), "Val(Sgnl)"=FALSE ("Value (Signaling)")) -> ()  [unwired: 2 in, 2 out]
          }
          frame True {
            n248 = property on="Finish Filling" class="Bool (strict)"("DisabledEnum"=T2."Enabled" ("Disabled")) -> ()  [unwired: 2 in, 2 out]
          }
        }
      }
      frame "Testing" {
        # "Require safety override if\nthere is a difference of\n>100psi across the valve"
        # "PT-2O - PT-IO"
        # "PT-1F - PT-IF"
        # "PT-1:2O"
        # "PT-1:2F"
        # "PT-3P - Ambient"
        # "PT - 2:3P"
        n249 = Array Subset(array=w357, index=13, length=3) -> (w359:dbl[])
        n250 = Array To Cluster(array=w359) -> (cluster=w358:T3)
        n251 = Unbundle(w358) -> ("[1]"=w324:dbl, "[2]"=w323:dbl)  [unwired: 7 out]
        n252 = Array Subset(array=w357, index=0, length=8) -> (w377:dbl[])
        n253 = Array To Cluster(array=w377) -> (cluster=w376:T3)
        n254 = Unbundle(w376) -> ("[0]"=w334:dbl, "[1]"=w325:dbl, "[3]"=w337:dbl, "[4]"=w338:dbl, "[7]"=w335:dbl, "[8]"=w336:dbl)  [unwired: 3 out]
        n255 = Subtract(x=w324, y=w323) -> (x-y=w364:dbl)
        n256 = Subtract(x=w323, y=14.0) -> (x-y=w356:dbl)
        n257 = Subtract(x=w337, y=w338) -> (x-y=w372:dbl)
        n258 = Subtract(x=w334, y=w325) -> (x-y=w352:dbl)
        n259 = Subtract(x=w337, y=w336) -> (x-y=w375:dbl)
        n260 = Subtract(x=w335, y=w325) -> (x-y=w367:dbl)
        n261 = Absolute Value(x=w364) -> (abs(x)=w363:dbl)
        n262 = Absolute Value(x=w367) -> (abs(x)=w366:dbl)
        n263 = Absolute Value(x=w356) -> (abs(x)=w355:dbl)
        n264 = Absolute Value(x=w352) -> (abs(x)=w369:dbl)
        n265 = Absolute Value(x=w375) -> (abs(x)=w374:dbl)
        n266 = Absolute Value(x=w372) -> (abs(x)=w371:dbl)
        n267 = Greater?(x=w369, y=100) -> (0:w341:bool)
        n268 = Greater?(x=w374, y=100) -> (0:w340:bool)
        n269 = Greater?(x=w366, y=100) -> (0:w339:bool)
        n270 = Greater?(x=w363, y=100) -> (0:w344:bool)
        n271 = Greater?(x=w371, y=100) -> (0:w342:bool)
        n272 = Greater?(x=w355, y=100) -> (0:w343:bool)
        n273 = Build Array(w344, w343, w342, w341, w340, w339) -> (w351:bool[])
        n274 = Compound Arithmetic op=OR(w333, w351, "Spark Safety") -> (invert w346:bool[])
        n275 = Or(x="Safety Override", y=w346) -> (x .or. y?=w347:bool[])
        n276 = Build Array("NC-P", "NO-P", "NC-F", "NC-O", "NC-IF", "NC-IO") -> (w326:T1[])
        n277 = And(x=w347, y=w326) -> (x .and. y?=w350:T1[])
        n278 = And(x="Spark Safety", y="Spark Test") -> (x .and. y?=w321:bool)
        n279 = Exclusive Or(1:w350, 2:w349) -> (0:w348:T1[])
      }
    }
    "Pump" <- w122
    "Ignition" <- w112
    n280 = feedback-in #3(w129) -> ()
    n281 = Or(x="F Purge", y=w83) -> (x .or. y?=w85:bool)
    n282 = Build Array("O Purge", w85) -> (w94:bool[])
    n283 = case shown="\"Abort\", \"Finished\"" w108 {
      tunnel: [FALSE w167 TRUE] -> w102
      tunnel: [FALSE w166 TRUE] -> w101
      tunnel: w100 -> [_ _ w171]
      tunnel: [bool[] [FALSE, FALSE, FALSE, FALSE, FALSE, FALSE, FALSE] bool[] [FALSE, FALSE, FALSE, FALSE, FALSE, FALSE, FALSE] w174] -> w96
      tunnel: w94 -> [_ _ w173]
      tunnel: w93 -> [_ w167 _]
      tunnel: w92 -> [_ w166 _]
      frame Default {
        n284 = property on="O Purge" class="Bool (strict)"("DisabledEnum"=2, "Value"=FALSE ("Ox Purge")) -> ()  [unwired: 2 in, 2 out]
        n285 = call "BtnColor.vi"("Selector"=0.0) -> ("Text Color"=w153:i32, "Colors"=w152:cluster{u32, u32}[], "Text"=w154:string, "Disabled"=w155:i32)  [unwired: 4 in]
        n286 = property on="ABORT" class="Bool"("DisabledEnum"=w155, "BoolText.Text"=w154, "Colors [4]"=w152, "BoolText.TextColor"=w153) -> ()  [unwired: 2 in, 2 out]
        n287 = property on="F Purge" class="Bool (strict)"("DisabledEnum"=2, "Value"=FALSE ("Fuel Purge")) -> ()  [unwired: 2 in, 2 out]
      }
      frame "Testing" {
        n288 = property on="O Purge" class="Bool (strict)"("Value"="Oxygen Purge") -> ()  [unwired: 2 in, 2 out]
        n289 = property on="F Purge" class="Bool (strict)"("Value"="Fuel Purge") -> ()  [unwired: 2 in, 2 out]
      }
      frame "Abort", "Finished" {
        w186 = FALSE
        n290 = property on="F Purge" class="Bool (strict)"("DisabledEnum"=0) -> ()  [unwired: 2 in, 2 out]
        n291 = property on="O Purge" class="Bool (strict)"("DisabledEnum"=0) -> ()  [unwired: 2 in, 2 out]
        n292 = And(x=w171, y="Depressurize") -> (x .and. y?=w185:bool)
        n293 = Select(t=2.0, s=w185, f=1.0) -> (s? t:f=w178:dbl)
        n294 = call "BtnColor.vi"("Selector"=w178) -> ("Text Color"=w175:i32, "Colors"=w176:cluster{u32, u32}[], "Text"=w177:string, "Disabled"=w179:i32)  [unwired: 4 in]
        n295 = property on="ABORT" class="Bool"("DisabledEnum"=w179, "BoolText.Text"=w177, "BoolText.TextColor"=w175, "Colors [4]"=w176) -> ()  [unwired: 2 in, 2 out]
        n296 = Or Array Elements(Boolean array=w173) -> (logical OR=w172:bool)
        n297 = Compound Arithmetic op=AND(invert w172, w171) -> (w170:bool)
        n298 = Select(t=0.0, s=w170, f=2.0) -> (s? t:f=w180:dbl)
        n299 = And(x="Depressurize", y=w170) -> (x .and. y?=w169:bool)
        n300 = property on="Depressurize" class="Bool (strict)"("DisabledEnum"=w180) -> ()  [unwired: 2 in, 2 out]
        n301 = Build Array(w186, w169, w186, w186, w186, w186) -> (w174:bool[])
      }
    }
    n302 = case shown="False" w109 {
      selector: w109 -> [w200 w225]
      tunnel: [w194 w216] -> w116
      tunnel: [w193 w215] -> w118
      tunnel: w115 -> [w198 w223]
      tunnel: w117 -> [w197 w222]
      tunnel: w111 -> [w192 w214]
      tunnel: w112 -> [_ w213]
      tunnel: w94 -> [w191 _]
      frame False {
        n303 = Not Equal?(x=w200, y=w192) -> (x != y?=w199:bool)
        n304 = case shown="True" w199 {
          tunnel: w198 -> [w201 w204]
          tunnel: w197 -> [w202 w203]
          tunnel: [w201 w210] -> w196
          tunnel: [w202 w207] -> w195
          frame False {
          }
          frame True {
            n305 = call <vilib>:"DAQmx Stop Task.vi"("task/channels in"=w204, "error in"=w203) -> ("task out"=w206:refnum<k21>, "error out"=w205:errorcluster)  [unwired: 12 in]
            n306 = call <vilib>:"DAQmx Clear Task.vi"("task in"=w206, "error in"=w205) -> ("error out"=w212:errorcluster)  [unwired: 13 in]
            n307 = call-poly <vilib>:"DAQmx Create Virtual Channel.vi"("lines"=tag "cDAQ1Mod2/port0/line1:2", "error in"=w212) -> ("task out"=w209:refnum<k21>, "error out"=w208:errorcluster)  [unwired: 12 in]
            n308 = call <vilib>:"DAQmx Start Task.vi"("task/channels in"=w209, "error in"=w208) -> ("task out"=w210:refnum<k21>, "error out"=w207:errorcluster)  [unwired: 12 in]
          }
        }
        n309 = call-poly <vilib>:"DAQmx Write.vi"("task/channels in"=w196, "data"=w191, "error in"=w195) -> ("task out"=w194:refnum<k21>, "error out"=w193:errorcluster)  [unwired: 10 in, 1 out]
      }
      frame True {
        # "State Change"
        # "Sparking"
        n310 = Not Equal?(x=w225, y=w214) -> (x != y?=w224:bool)
        n311 = case shown="True" w224 {
          tunnel: [w233 w241] -> w215
          tunnel: [w234 w240] -> w216
          tunnel: w223 -> [w234 w236]
          tunnel: w222 -> [w233 w235]
          frame False {
          }
          frame True {
            w244 = 10373 items=["Hz"=10373] ("units")
            w246 = 10307 items=["Pulse"=10265, "Toggle"=10307] ("CtrOutEvent.OutputBehavior")
            w252 = 10123 items=["Finite Samples"=10178, "Continuous Samples"=10123, "Hardware Timed Single Point"=12522] ("sample mode")
            w254 = 10214 items=["High"=10192, "Low"=10214] ("idle state")
            # "Initialization of spark plug waveform. Dwell time of 3 ms in a 20% duty cycle."
            n312 = call <vilib>:"DAQmx Stop Task.vi"("task/channels in"=w236, "error in"=w235) -> ("task out"=w238:refnum<k21>, "error out"=w237:errorcluster)  [unwired: 12 in]
            n313 = call <vilib>:"DAQmx Clear Task.vi"("task in"=w238, "error in"=w237) -> ("error out"=w239:errorcluster)  [unwired: 13 in]
            n314 = call-poly <vilib>:"DAQmx Create Virtual Channel.vi"("frequency"=66.6666, "duty cycle"=0.8, "counter"=tag "cDAQ1Mod2/ctr0", "units"=w244, "error in"=w239, "idle state"=w254, "initial delay"=0.0) -> ("task out"=w250:refnum<k21>, "error out"=w249:errorcluster)  [unwired: 7 in]
            n315 = property class="DAQmx Export Signal"(reference=w250, error in=w249, "Events:Counter Output Event:Output Terminal"=tag "/cDAQ1Mod2/PFI0" ("CtrOutEvent.OutputTerm"), "Events:Counter Output Event:Output Behavior"=w246) -> (reference out=w248:refnum<k21>, error out=w247:errorcluster)
            n316 = call-poly <vilib>:"DAQmx Timing.vi"("task/channels in"=w248, "sample mode"=w252, "error in"=w247) -> ("task out"=w240:refnum<k21>, "error out"=w241:errorcluster)  [unwired: 11 in]
          }
        }
        n317 = call <vilib>:"DAQmx Is Task Done.vi"("task/channels in"=w216, "error in"=w215) -> ("task out"=w221:refnum<k21>, "task done?"=w217:bool, "error out"=w220:errorcluster)  [unwired: 11 in]
        n318 = Not(x=w217) -> (.not. x?=w218:bool)
        n319 = Exclusive Or(1:w218, 2:w213) -> (0:w219:bool)
        n320 = case shown="True" w219 {
          tunnel: w221 -> [_ w228]
          tunnel: w220 -> [_ w227]
          tunnel: w213 -> [_ w226]
          frame False {
          }
          frame True {
            n321 = case shown="False" w226 {
              tunnel: w228 -> [w230 w232]
              tunnel: w227 -> [w229 w231]
              frame False {
                n322 = call <vilib>:"DAQmx Stop Task.vi"("task/channels in"=w230, "error in"=w229) -> ()  [unwired: 12 in, 2 out]
              }
              frame True {
                n323 = call <vilib>:"DAQmx Start Task.vi"("task/channels in"=w232, "error in"=w231) -> ()  [unwired: 12 in, 2 out]
              }
            }
          }
        }
      }
    }
    n324 = feedback-in #5(w116) -> ()
    n325 = feedback-in #6(w118) -> ()
    n326 = And(x=w93, y=w102) -> (x .and. y?=w106:bool)
    n327 = And(x=w92, y=w101) -> (x .and. y?=w105:bool)
    n328 = Or(x=w106, y="O Purge") -> (x .or. y?=w107:bool)
    "Ox Purged" <- w107
    n329 = Or(x=w105, y="F Purge") -> (x .or. y?=w104:bool)
    "Fuel Purged" <- w104
    n330 = feedback-in #7(w104) -> ()
    n331 = feedback-in #8(w107) -> ()
    n332 = Replace Array Subset(array=w96, new element=w85, index=0) -> (w95:bool[])
    n333 = Or(x=w98, y=w95) -> (x .or. y?=w99:T1[])
    n334 = call "SolenoidSignalBuilder.vi"("Solenoid Status"=w99, "Pump Status"=w122) -> ("NI9401_1 Signals"=w123:bool[])  [unwired: 6 in]
    "Solenoid\nStatus" <- w123
    n335 = call "NI9401_1"("data"=w123) -> ()  [unwired: 17 in, 2 out]
    n336 = feedback-in #9(w135) -> ()
  }
